vi "LVPong_main.vi"() -> ()   [LabVIEW 8.6]
uses:
  VI_Control/GameStatus Ctrl.ctl
  <vilib>/Utility/miscctls.llb/LVPositionTypeDef.ctl
  VI_Control/Ball Center Ctrl.ctl
panel:
  out "Direction":cluster{"x_dir":i32, "y_dir":i32}
  out "cheat":bool
  out "total_stg":i32
  in  "Ball":bool
  out "Gmsg":string
  in  "Brick 36":bool
  in  "Brick 35":bool
  in  "Brick 34":bool
  in  "Brick 33":bool
  in  "Brick 32":bool
  in  "Brick 31":bool
  in  "Brick 30":bool
  in  "Brick 29":bool
  in  "Brick 28":bool
  in  "Brick 27":bool
  in  "Brick 26":bool
  in  "Brick 25":bool
  out "Stage":i32
  out "shoot":bool
  in  "Paddle":bool
  out "Position":T1
  out "Ball Center":T2
  in  "stop":bool
  out "COMBO":i32
  out "SCORE":i32
  out "LIVE":i16
  in  "Brick 24":bool
  in  "Brick 23":bool
  in  "Brick 22":bool
  in  "Brick 21":bool
  in  "Brick 20":bool
  in  "Brick 19":bool
  in  "Brick 18":bool
  in  "Brick 17":bool
  in  "Brick 16":bool
  in  "Brick 15":bool
  in  "Brick 14":bool
  in  "Brick 13":bool
  in  "Brick 12":bool
  in  "Brick 11":bool
  in  "Brick 10":bool
  in  "Brick 9":bool
  in  "Brick 8":bool
  in  "Brick 7":bool
  in  "Brick 6":bool
  in  "Brick 5":bool
  in  "Brick 4":bool
  in  "Brick 3":bool
  in  "Brick 2":bool
  in  "Brick 1":bool
  # "基本雙迴圈同步功能演示\n複合鍵觸發EVENT演示\n物件Method和property展示\n碰撞演算法是AABB檢測加四個角的距離檢測\n沒有使用分離軸法"
  # "by hls Ver1.1"
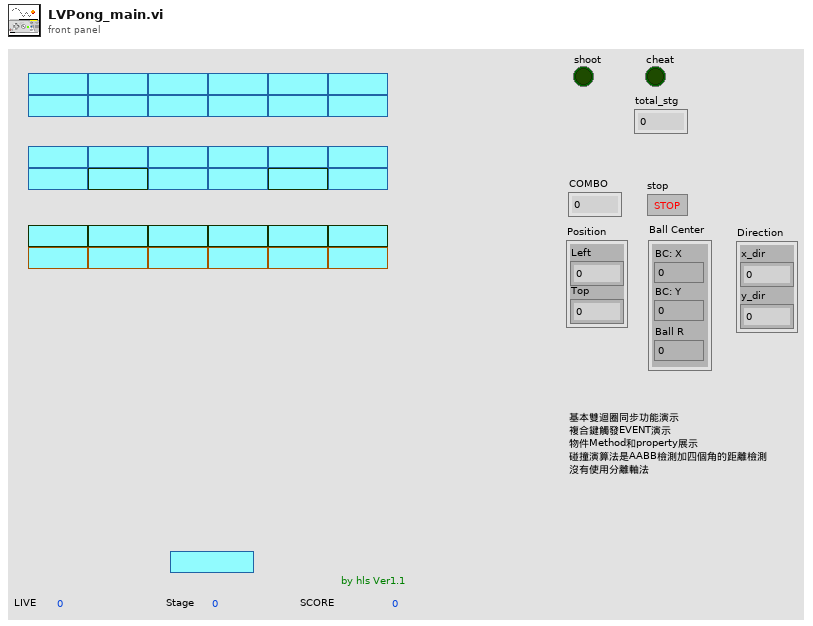
[diagram p1: front panel]
types:
  T1 = typedef "LVPositionTypeDef.ctl" = cluster{"Left":i32, "Top":i32}
  T2 = typedef "Ball Center Ctrl.ctl" = cluster{"BC: X":i32, "BC: Y":i32, "Ball R":i32}
  T3 = typedef "GameStatus Ctrl.ctl" = enum16{"set_stg", "wait", "running", "clear", "end"}
  T4 = typedef "LVBoundsTypeDef.ctl" = cluster{"Width":u32, "Height":u32}
  T5 = cluster{"Left":i32, "Right":i32, "Top":i32, "Bottom":i32, "Center_x":i32, "Center_y":i32, "R":i32}
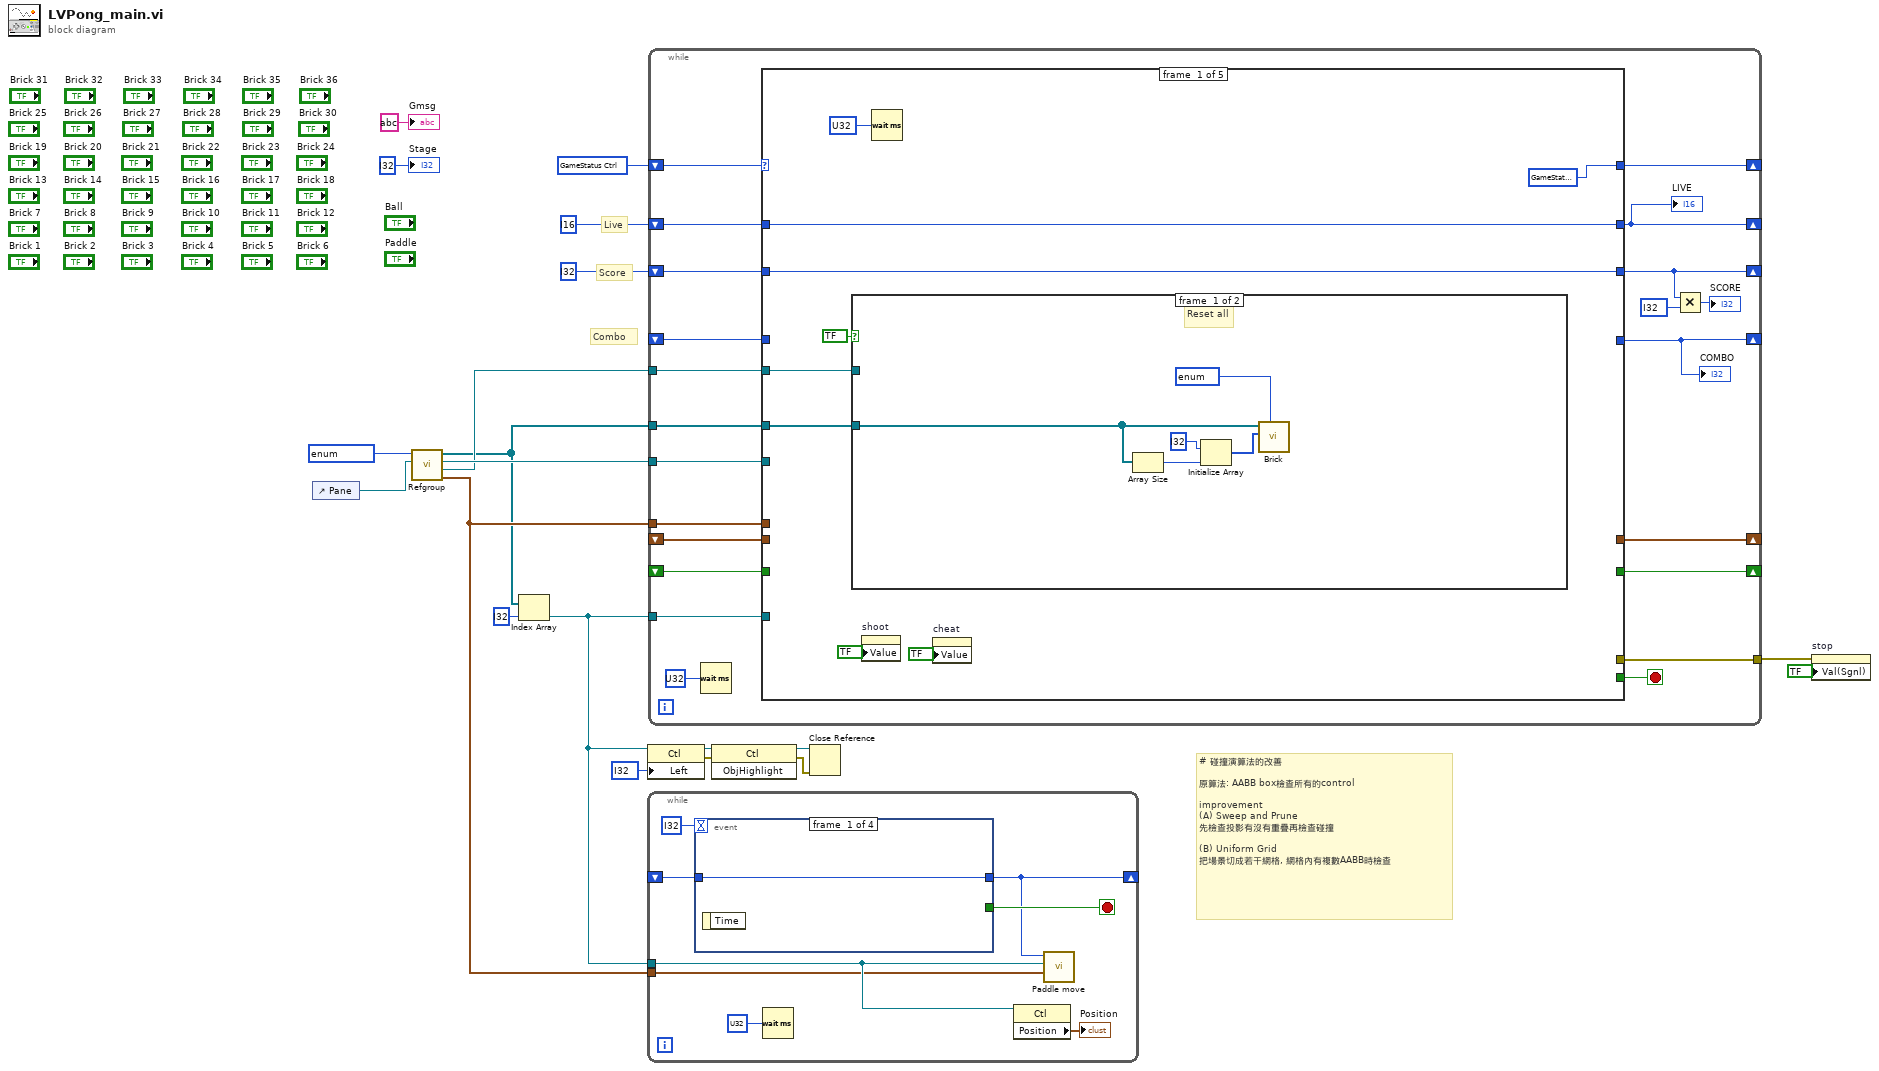
[diagram p0: block diagram]
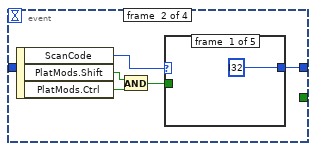
[diagram p2: hidden frame]
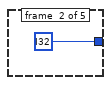
[diagram p3: hidden frame]
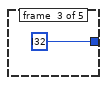
[diagram p4: hidden frame]
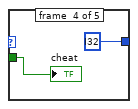
[diagram p5: hidden frame]
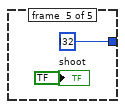
[diagram p6: hidden frame]
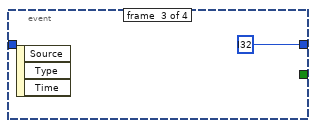
[diagram p7: hidden frame]
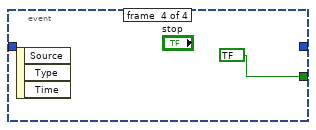
[diagram p8: hidden frame]
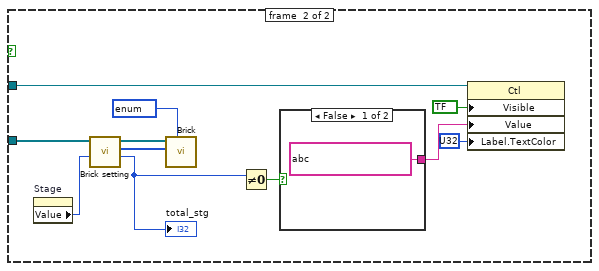
[diagram p9: hidden frame]
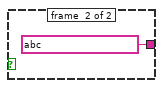
[diagram p10: hidden frame]
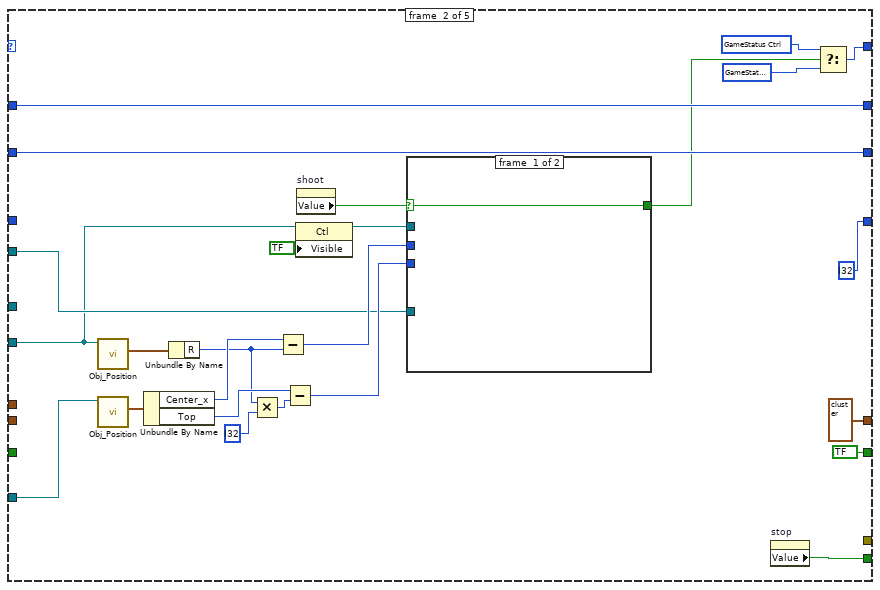
[diagram p11: hidden frame]
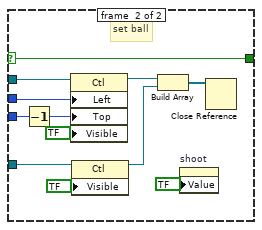
[diagram p12: hidden frame]
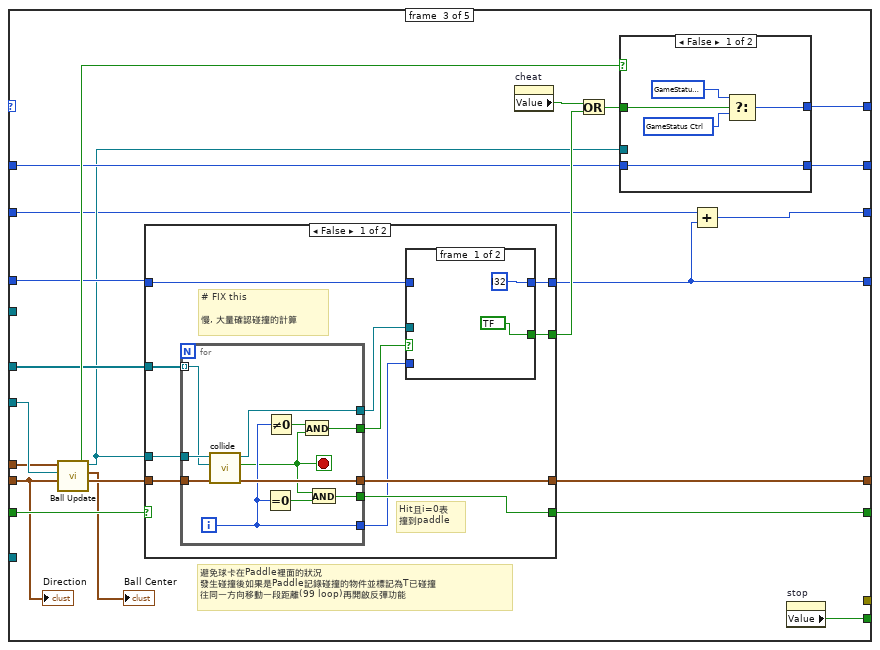
[diagram p13: hidden frame]
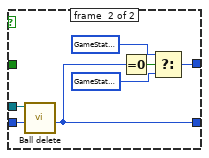
[diagram p14: hidden frame]
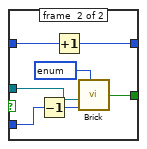
[diagram p15: hidden frame]
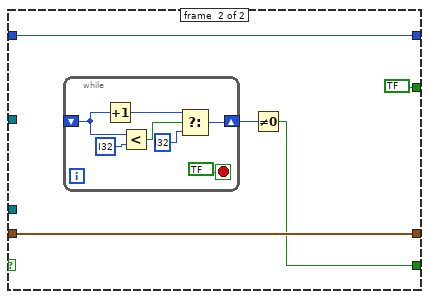
[diagram p16: hidden frame]
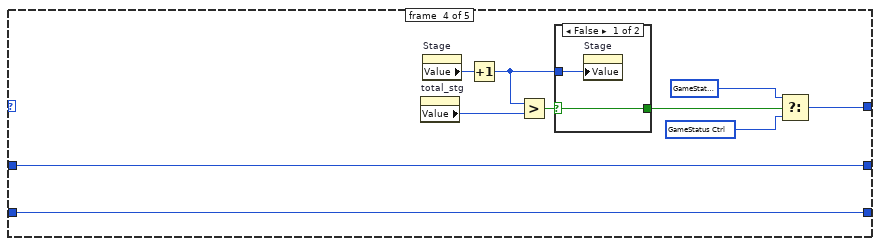
[diagram p17: hidden frame]
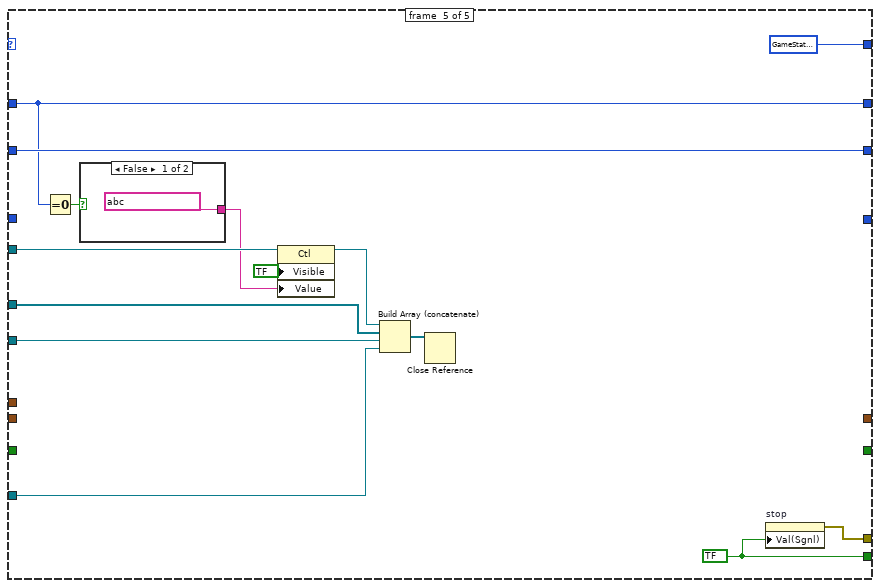
[diagram p19: hidden frame]
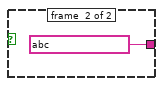
[diagram p20: hidden frame]
diagram:
  # "# 碰撞演算法的改善\n\n原算法: AABB box檢查所有的control\n\nimprovement\n(A) Sweep and Prune\n先檢查投影有沒有重疊再檢查碰撞\n\n(B) Uniform Grid\n把場景切成若干網格, 網格內有複數AABB時檢查"
  # "Combo"
  # "Score"
  # "Live"
  n1 = control-ref of="Pane"() -> (w14:refnum<vi>)
  n2 = call "Refgroup.vi"("Pane"=w14, "Action"=enum16{"GetRef", "ChkRef"} ?) -> ("AreaSize"=w12:T4, "Ref_Gmsg"=w10:refnum<vi>, "Ref_Ball"=w11:refnum<vi>, "Ref_brick"=w1:refnum<vi>[])  [unwired: 2 in]
  n3 = Index Array(array=w1, index=i32 ?) -> (element=w7:refnum<vi>)
  n4 = property class="Ctl"(reference=w7, "Left"=i32 ? ("Position:Left")) -> (reference out=w5:refnum<vi>, error out=w4:errorcluster)  [unwired: 1 in]
  n5 = while {
    shift-right: [w22] -> _
    shift-left: _ -> [w27]
    tunnel: w7 -> [w25]
    tunnel: w12 -> [w21]
    stop <- w23 stop-if-true
    n6 = event shown="[3] \"stop\": Value Change" {
      selector: _ -> [_ _ _ _]
      dyn-events: _ -> [_ _ _ _]
      timeout: i32 ? -> [_ _ _ _]
      tunnel: [_ _ _ bool ? ("stop")] -> w23
      tunnel: [w29 w34 i32 ? _] -> w22
      tunnel: w27 -> [w29 _ _ _]
      event #0 {
        n7 = event-data() -> ()  [unwired: 1 in, 1 out]
      }
      event #1 {
        n8 = event-data() -> ("ScanCode"=w33:i16, "PlatMods.Shift"=w31:bool, "PlatMods.Ctrl"=w32:bool)  [unwired: 1 in]
        n9 = And(x=w31, y=w32) -> (x .and. y?=w30:bool)
        n10 = case shown="77" w33 {
          tunnel: [i32 ? i32 ? i32 ? i32 ? i32 ?] -> w34
          tunnel: w30 -> [_ _ _ w38 _]
          frame #0 {
          }
          frame #1 {
          }
          frame #2 {
          }
          frame #3 {
            "cheat" <- w38
          }
          frame #4 {
            "shoot" <- bool ?
          }
        }
      }
      event #2 {
        n11 = event-data() -> ()  [unwired: 1 in, 3 out]
      }
      event #3 {
        n12 = event-data() -> ()  [unwired: 1 in, 3 out]
      }
    }
    n13 = Wait (ms)(milliseconds to wait=u32 ? ("speed")) -> ()  [unwired: 1 out]
    n14 = property class="Ctl"(reference=w25) -> ("Position"=→"Position":T1)  [unwired: 1 in, 2 out]
    n15 = call "Paddle move.vi"("AreaSize"=w21, "Paddle Ref"=w25, "offset"=w22) -> ()  [unwired: 4 in, 1 out]
  }
  n16 = while {
    shift-right: [w63] -> _
    shift-left: _ -> [w65]
    tunnel: w1 -> [w62]
    shift-right: [w44] -> _
    shift-left: _ -> [w61]
    shift-right: [w48] -> _
    shift-left: i16 ? ("Ball") -> [w51]
    shift-right: [w45] -> _
    shift-left: i32 ? ("Sc") -> [w57]
    shift-right: [w58] -> _
    shift-left: T3 ? -> [w59]
    shift-right: [w56] -> _
    shift-left: _ -> [w55]
    tunnel: w7 -> [w54]
    tunnel: w11 -> [w53]
    tunnel: [w52] -> w16
    tunnel: w12 -> [w50]
    tunnel: w10 -> [w49]
    stop <- w60 stop-if-true
    n17 = Wait (ms)(milliseconds to wait=u32 ? ("speed")) -> ()  [unwired: 1 out]
    n18 = case shown="\"running\"" w59 {
      tunnel: w65 -> [_ _ w141 _ _]
      tunnel: [_ cluster{"x_dir":i32, "y_dir":i32} ? ("Direction") w150 _ _] -> w63
      tunnel: w62 -> [w71 _ w138 _ w224]
      tunnel: w61 -> [_ _ w136 _ _]
      tunnel: [_ i32 ? w134 _ _] -> w44
      tunnel: [_ w112 w145 _ w232] -> w60
      tunnel: w51 -> [w72 w117 w133 w208 w230]
      tunnel: [w72 w117 w137 w208 w230] -> w48
      tunnel: w57 -> [w69 w97 w131 w213 w233]
      tunnel: [w69 w97 w152 w213 w233] -> w45
      tunnel: [T3 ? w113 w151 w215 T3 ?] -> w58
      tunnel: [_ bool ? ("Hit") w140 _ _] -> w56
      tunnel: w55 -> [_ _ w149 _ _]
      tunnel: w54 -> [_ w109 _ _ w222]
      tunnel: w53 -> [_ w93 w148 _ w223]
      tunnel: [_ _ _ _ w231] -> w52
      tunnel: w50 -> [_ _ w147 _ _]
      tunnel: w49 -> [w70 w94 _ _ w229]
      frame #0 {
        n19 = case shown="True" bool ? {
          tunnel: w71 -> [w77 w85]
          tunnel: w70 -> [_ w87]
          frame #0 {
            # "Reset all"
            n20 = Array Size(array=w77) -> (size(s)=w76:i32)
            n21 = Initialize Array(i32 ? ("element"), w76) -> (w75:i32[])
            n22 = call "Brick.vi"("Brick Ref table"=w77, "HP set"=w75, "Action"=enum16{"Hit", "Set"} ?) -> ()  [unwired: 4 in, 1 out]
          }
          frame #1 {
            n23 = property on="Stage" class="DigNum (strict)"() -> ("Value"=w81:i32)  [unwired: 2 in, 2 out]
            n24 = call "Brick setting.vi"("stage"=w81, "Ref_brick"=w85) -> ("total_stg"=w82:i32, "HP set"=w86:i32[], "Brick_table"=w84:refnum<vi>[])  [unwired: 2 in, 1 out]
            "total_stg" <- w82
            n25 = call "Brick.vi"("Brick Ref table"=w84, "HP set"=w86, "Action"=enum16{"Hit", "Set"} ?) -> ()  [unwired: 4 in, 1 out]
            n26 = Not Equal To 0?(x=w82) -> (x != 0?=w83:bool)
            n27 = case shown="False" w83 {
              tunnel: [string ? string ?] -> w89
              frame #0 {
              }
              frame #1 {
              }
            }
            n28 = property class="Ctl"(reference=w87, "Visible"=bool ?, "Value"=w89, "Label.TextColor"=u32 ? ("Label.Text Colors:Text Color")) -> ()  [unwired: 1 in, 2 out]
          }
        }
        n29 = property on="shoot" class="Bool (strict)"("Value"=bool ? ("123")) -> ()  [unwired: 2 in, 2 out]
        n30 = Wait (ms)(milliseconds to wait=u32 ? ("speed")) -> ()  [unwired: 1 out]
        n31 = property on="cheat" class="Bool (strict)"("Value"=bool ? ("cheat")) -> ()  [unwired: 2 in, 2 out]
      }
      frame #1 {
        n32 = call "Obj_Position.vi"("Ctl Refnum"=w93) -> ("Position"=w107:T5)  [unwired: 5 in, 1 out]
        n33 = call "Obj_Position.vi"("Ctl Refnum"=w109) -> ("Position"=w108:T5)  [unwired: 5 in, 1 out]
        n34 = Unbundle By Name(w108) -> ("Center_x"=w106:i32, "Top"=w105:i32)
        n35 = Unbundle By Name(w107) -> ("R"=w103:i32)
        n36 = Multiply(x=w103, y=i32 ?) -> (x*y=w104:i32)
        n37 = Subtract(x=w106, y=w103) -> (x-y=w101:i32)
        n38 = Subtract(x=w105, y=w104) -> (x-y=w100:i32)
        n39 = property class="Ctl"(reference=w93, "Visible"=bool ?) -> (reference out=w99:refnum<vi>)  [unwired: 1 in, 1 out]
        n40 = property on="shoot" class="Bool (strict)"() -> ("Value"=w110:bool)  [unwired: 2 in, 2 out]
        n41 = case shown="True" w110 {
          selector: w110 -> [w118 w125]
          tunnel: w94 -> [_ w130]
          tunnel: w99 -> [_ w128]
          tunnel: w101 -> [_ w127]
          tunnel: w100 -> [_ w120]
          tunnel: [w118 w125] -> w95
          frame #0 {
          }
          frame #1 {
            # "set ball"
            n42 = Decrement(x=w120) -> (x-1=w119:i32)
            n43 = property class="Ctl"(reference=w128, "Left"=w127, "Top"=w119, "Visible"=bool ?) -> (reference out=w123:refnum<vi>)  [unwired: 1 in, 1 out]
            n44 = property class="Ctl"(reference=w130, "Visible"=bool ?) -> (reference out=w122:refnum<vi>)  [unwired: 1 in, 1 out]
            n45 = Build Array(w123, w122) -> (w121:refnum<vi>[])
            n46 = property on="shoot" class="Bool (strict)"("Value"=bool ? ("123")) -> ()  [unwired: 2 in, 2 out]
            n47 = Close Reference(reference=w121) -> ()  [unwired: 1 in, 1 out]
          }
        }
        n48 = property on="stop" class="Bool (strict)"() -> ("Value"=w112:bool)  [unwired: 2 in, 2 out]
        n49 = Select(t=T3 ?, s=w95, f=T3 ?) -> (s? t:f=w113:T3)
      }
      frame #2 {
        # "避免球卡在Paddle裡面的狀況\n發生碰撞後如果是Paddle記錄碰撞的物件並標記為T已碰撞\n往同一方向移動一段距離(99 loop)再開啟反彈功能"
        n50 = call "Ball Update.vi"("Direction in"=w141, "Ball Ref"=w148, "AreaSize"=w147) -> ("LostBall"=w144:bool, "Direction"=w146:cluster{"x_dir":i32, "y_dir":i32}, "Ball Center"=→"Ball Center":T2, "Ball ref out"=w132:refnum<vi>)  [unwired: 1 in]
        n51 = case shown="False" w149 {
          tunnel: w146 -> [w175 w200]
          tunnel: w138 -> [w174 _]
          tunnel: w132 -> [w173 _]
          tunnel: [w172 w200] -> w150
          tunnel: [w171 w199] -> w140
          tunnel: w136 -> [w167 w197]
          tunnel: [w166 bool ? ("Brick set")] -> w135
          tunnel: [w165 w197] -> w134
          frame #0 {
            # "# FIX this\n\n慢, 大量確認碰撞的計算"
            # "Hit且i=0表\n撞到paddle"
            n52 = for {
              tunnel: w173 -> [w194]
              tunnel: [w192] -> w172
              tunnel: w174 -> [w193] mode=indexing
              tunnel: w175 -> [w195]
              tunnel: [w191] -> w168
              tunnel: [w189] -> w170
              tunnel: [w187] -> w169
              tunnel: [w190] -> w171
              i -> [w187]
              stop <- w186 stop-if-true
              n53 = call "collide.vi"("Direction in"=w195, "Brick Ref"=w193, "Ball Ref"=w194) -> ("Direction"=w192:cluster{"x_dir":i32, "y_dir":i32}, "Hit"=w186:bool, "Brick out"=w189:refnum<vi>)  [unwired: 2 in]
              n54 = Equal To 0?(x=w187) -> (x = 0?=w185:bool)
              n55 = Not Equal To 0?(x=w187) -> (x != 0?=w188:bool)
              n56 = And(x=w188, y=w186) -> (x .and. y?=w191:bool)
              n57 = And(x=w186, y=w185) -> (x .and. y?=w190:bool)
            }
            n58 = case shown="True" w168 {
              tunnel: w167 -> [_ w184]
              tunnel: [i32 ? w182] -> w165
              tunnel: [bool ? w180] -> w166
              tunnel: w170 -> [_ w181]
              tunnel: w169 -> [_ w179]
              frame #0 {
              }
              frame #1 {
                n59 = Decrement(x=w179) -> (x-1=w178:i32)
                n60 = Increment(x=w184) -> (x+1=w182:i32)
                n61 = call "Brick.vi"("Hit Ref"=w181, "Brick_ind"=w178, "Action"=enum16{"Hit", "Set"} ?) -> ("Brick set"=w180:bool)  [unwired: 4 in]
              }
            }
          }
          frame #1 {
            n62 = while {
              shift-right: [w201] -> w198
              shift-left: _ -> [w205]
              stop <- bool ? stop-if-true
              n63 = Increment(x=w205) -> (x+1=w204:i32)
              n64 = Less?(x=w205, y=i32 ?) -> (x < y?=w203:bool)
              n65 = Select(t=w204, s=w203, f=i32 ?) -> (s? t:f=w201:i32)
            }
            n66 = Not Equal To 0?(x=w198) -> (x != 0?=w199:bool)
          }
        }
        n67 = property on="cheat" class="Bool (strict)"() -> ("Value"=w142:bool)  [unwired: 2 in, 2 out]
        n68 = Or(x=w142, y=w135) -> (x .or. y?=w143:bool)
        n69 = case shown="False" w144 {
          tunnel: [w157 w163] -> w151
          tunnel: w133 -> [w153 w160]
          tunnel: w143 -> [w154 _]
          tunnel: [w153 w158] -> w137
          tunnel: w132 -> [_ w159]
          frame #0 {
            n70 = Select(t=T3 ?, s=w154, f=T3 ?) -> (s? t:f=w157:T3)
          }
          frame #1 {
            n71 = call "Ball delete.vi"("ball hp"=w160, "Ball Ref"=w159) -> ("hp new"=w158:i16)  [unwired: 4 in, 1 out]
            n72 = Equal To 0?(x=w158) -> (x = 0?=w161:bool)
            n73 = Select(t=T3 ?, s=w161, f=T3 ?) -> (s? t:f=w163:T3)
          }
        }
        n74 = Add(x=w131, y=w134) -> (x+y=w152:i32)
        n75 = property on="stop" class="Bool (strict)"() -> ("Value"=w145:bool)  [unwired: 2 in, 2 out]
        "Direction" <- w141
      }
      frame #3 {
        n76 = property on="total_stg" class="DigNum (strict)"() -> ("Value"=w212:i32)  [unwired: 2 in, 2 out]
        n77 = property on="Stage" class="DigNum (strict)"() -> ("Value"=w214:i32)  [unwired: 2 in, 2 out]
        n78 = Increment(x=w214) -> (x+1=w210:i32)
        n79 = Greater?(x=w210, y=w212) -> (0:w211:bool)
        n80 = case shown="False" w211 {
          selector: w211 -> [w219 w220]
          tunnel: [w219 w220] -> w209
          tunnel: w210 -> [w218 _]
          frame #0 {
            n81 = property on="Stage" class="DigNum (strict)"("Value"=w218) -> ()  [unwired: 2 in, 2 out]
          }
          frame #1 {
          }
        }
        n82 = Select(t=T3 ?, s=w209, f=T3 ?) -> (s? t:f=w215:T3)
      }
      frame #4 {
        w232 = bool ?
        n83 = Equal To 0?(x=w230) -> (x = 0?=w226:bool)
        n84 = case shown="False" w226 {
          tunnel: [string ? string ?] -> w227
          frame #0 {
          }
          frame #1 {
          }
        }
        n85 = property class="Ctl"(reference=w229, "Visible"=bool ?, "Value"=w227) -> (reference out=w225:refnum<vi>)  [unwired: 1 in, 1 out]
        n86 = Build Array (concatenate)(w225, w224, w223, w222) -> (w221:refnum<vi>[])
        n87 = Close Reference(reference=w221) -> ()  [unwired: 1 in, 1 out]
        n88 = property on="stop" class="Bool (strict)"("Val(Sgnl)"=w232) -> (error out=w231:errorcluster)  [unwired: 2 in, 1 out]
      }
    }
    "LIVE" <- w48
    "COMBO" <- w44
    n89 = Multiply(x=w45, y=i32 ?) -> (x*y=→"SCORE":i32)
  }
  n90 = invoke class="Ctl" method="ObjHighlight"(reference=w5, error in=w4) -> (reference out=w2:refnum<vi>, error out=w3:errorcluster)  [unwired: 1 in, 1 out]
  n91 = Close Reference(reference=w2, error in (no error)=w3) -> ()  [unwired: 1 out]
  n92 = property on="stop" class="Bool (strict)"(error in=w16, "Val(Sgnl)"=bool ? ("Value (Signaling)")) -> ()  [unwired: 1 in, 2 out]
  "Gmsg" <- string ?
  "Stage" <- i32 ? ("Stage")
